vi "timer.vi"(8 "error in (no error)":errorcluster) -> (0 "error out":errorcluster, 2 "millisecond timer value":u32)   [LabVIEW 2017]
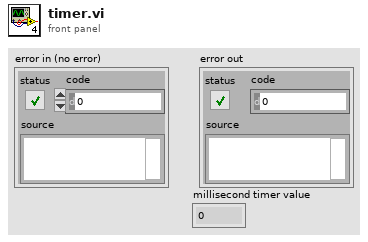
[diagram p1: front panel]
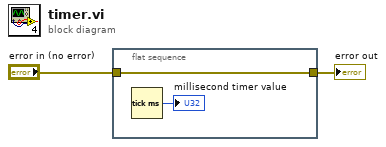
[diagram p0: block diagram]
diagram:
  n1 = flat-sequence {
    tunnel: [w4] -> w2
    tunnel: "error in (no error)" -> [w4]
    frame #0 {
      n2 = Tick Count (ms)() -> (millisecond timer value=→"millisecond timer value":u32)
    }
  }
  "error out" <- w2
